vi "SetMotors_ReadEncoders.vi"(4 "Reset Encoder 4":bool, 5 "Motor 1 speed":dbl(slide) scale=-100.0..100.0, 6 "Reset Encoder 3":bool, 7 "Motor 2 speed":dbl(slide) scale=-100.0..100.0, 8 "Reset Encoder 2":bool, 9 "Reset Encoder 1":bool, 10 "Motor 3 speed":dbl(slide) scale=-100.0..100.0, 11 "Motor 4 speed":dbl(slide) scale=-100.0..100.0) -> (0 "Counter 4":i32, 1 "Counter 3":i32, 2 "Counter 2":i32, 3 "Counter 1":i32)   [LabVIEW 2018]
panel:
  out "Motor 1 CM 2":dbl
  out "Motor 3 CM":dbl
  out "Motor 2 CM":dbl
  out "Motor 1 CM":dbl
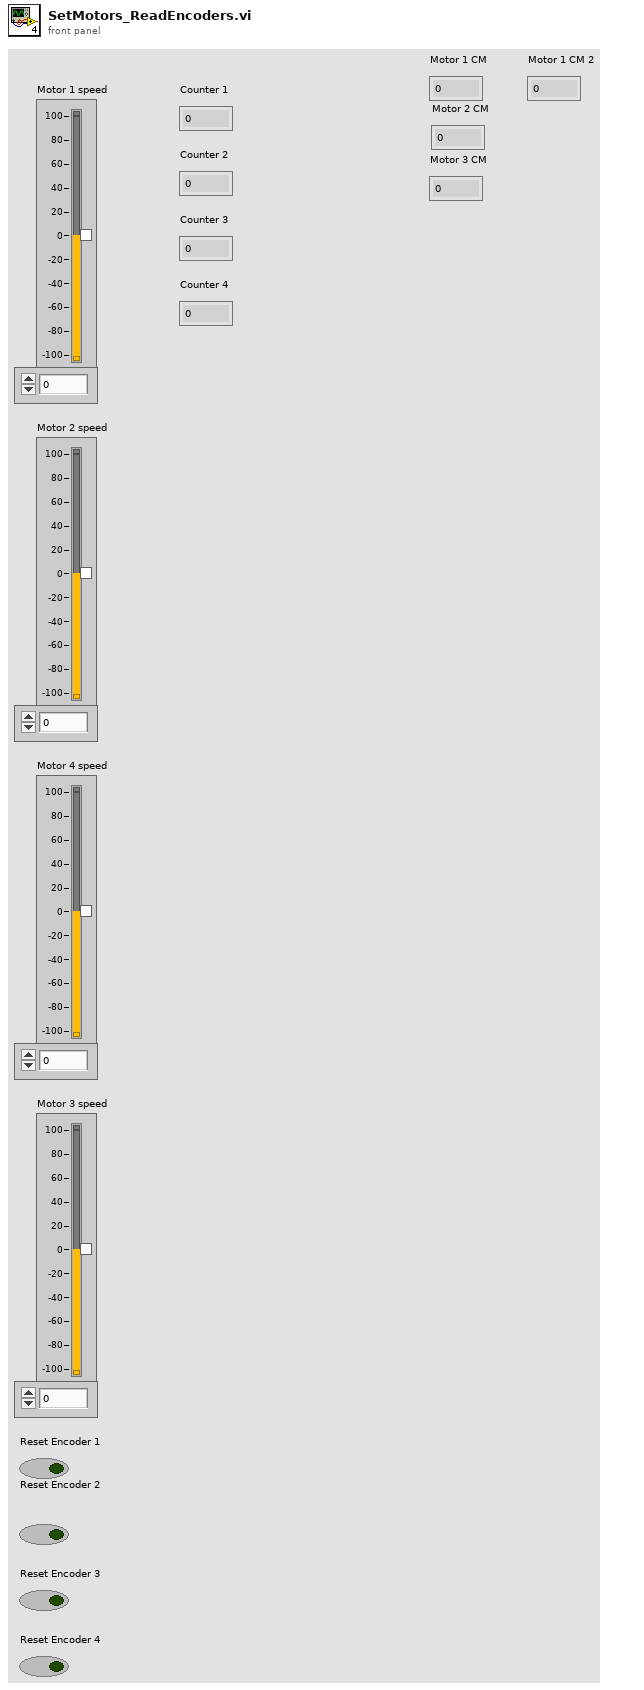
[diagram p1: front panel]
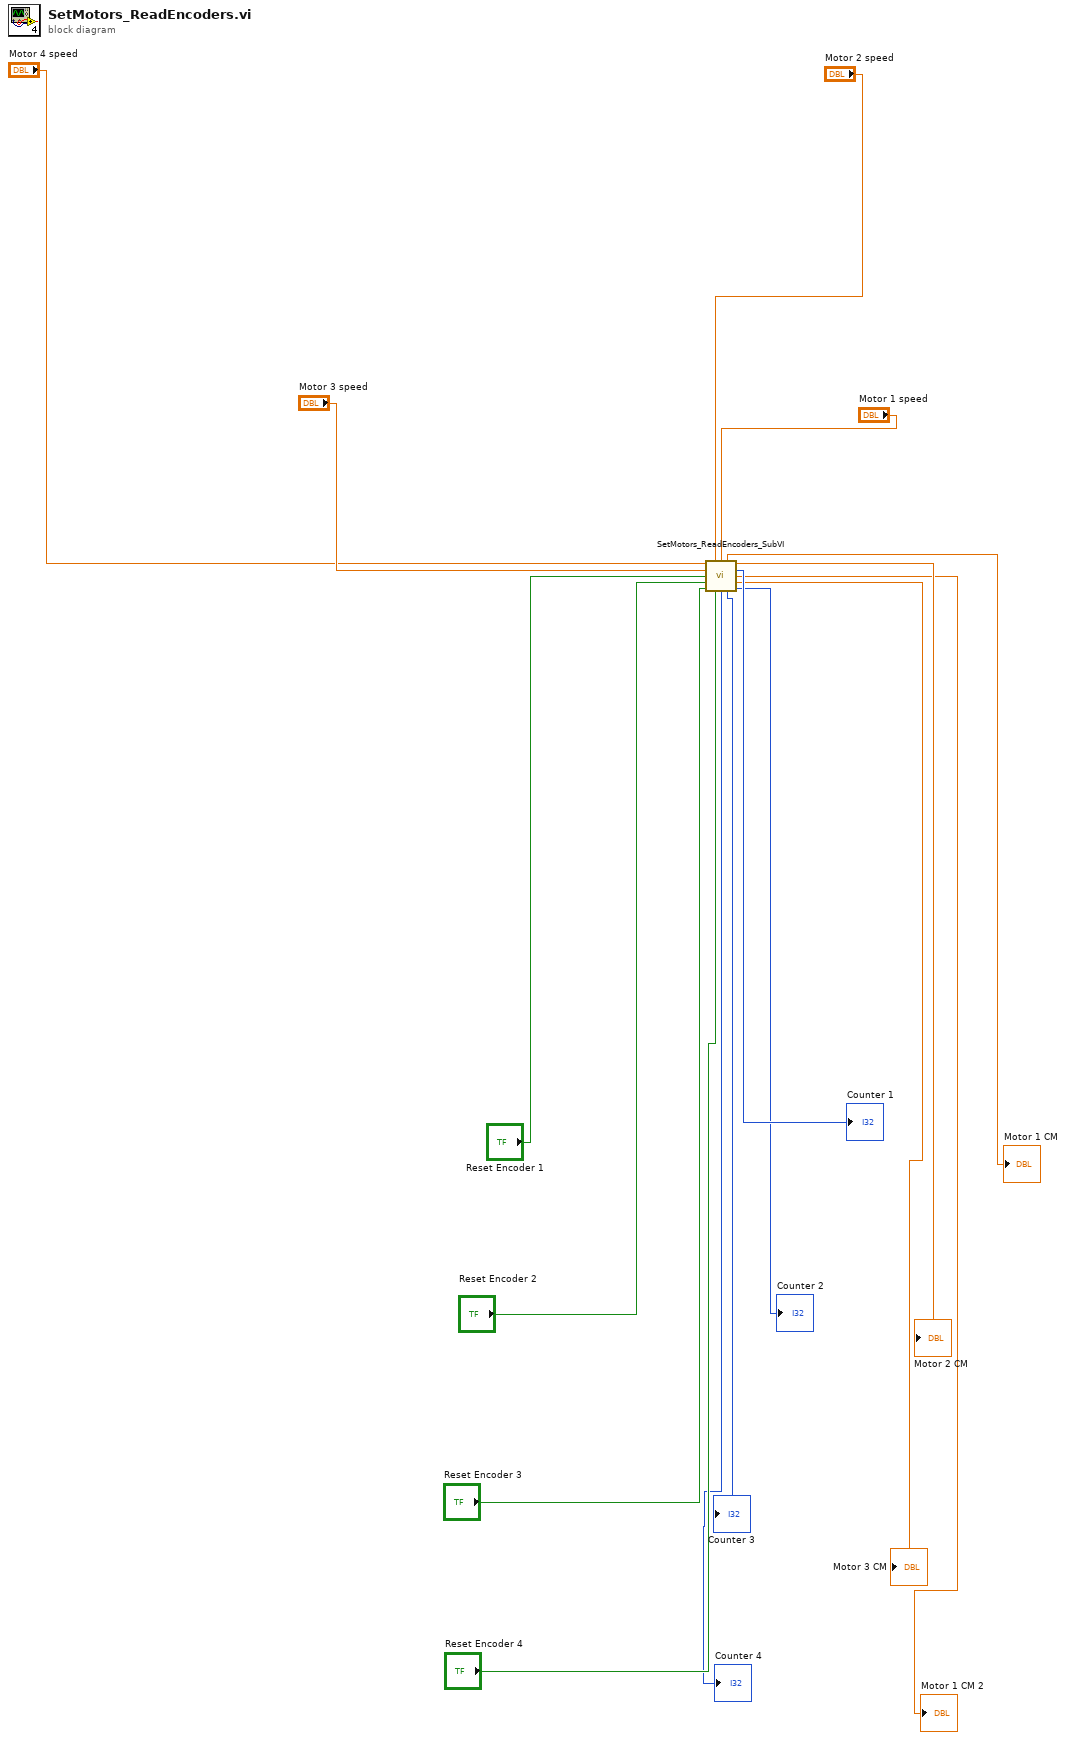
[diagram p0: block diagram]
diagram:
  n1 = call "SetMotors_ReadEncoders_SubVI.vi"("Motor 4 speed"="Motor 4 speed", "Motor 2 speed"="Motor 2 speed", "Motor 1 speed"="Motor 1 speed", "Motor 3 speed"="Motor 3 speed", "Reset Encoder 1"="Reset Encoder 1", "Reset Encoder 2"="Reset Encoder 2", "Reset Encoder 3"="Reset Encoder 3", "Reset Encoder 4"="Reset Encoder 4") -> ("Motor 1 CM"=→"Motor 1 CM":dbl, "Motor 2 CM"=→"Motor 2 CM":dbl, "Counter 1"=→"Counter 1":i32, "Motor 4 CM"=→"Motor 1 CM 2":dbl, "Motor 3 CM"=→"Motor 3 CM":dbl, "Counter 4"=→"Counter 4":i32, "Counter 3"=→"Counter 3":i32, "Counter 2"=→"Counter 2":i32)
